vi "EN50160 Aggregation 10min.vi"(0 "voltage RMS values":dbl[](array[numeric]), 1 "fundamental voltage unbalance u2 [%]":dbl, 2 "voltage THD [%]":dbl[](array[numeric]), 3 "harmonic subgroups complex spectra":cluster{"f0":dbl, "df":dbl, "vectors":cdb[]}[](array[cluster]), 4 "system info in":refnum<class "EP System Info.lvclass">, 5 "error in (no error)":errorcluster, 6 "reset? (F)":bool, 7 "voltage flags? (F)":bool[](array[boolean]), 8 "data timestamp":timestamp) -> (14 "10min values":T1, 18 "system info out":refnum<class "EP System Info.lvclass">, 19 "error out":errorcluster)   [LabVIEW 2014, in "NI_EP_Power Quality.lvlib"]
doc: "Calculates aggregated values of power quality parameters for specific intervals. You use the aggregated values for further evaluations according to EN 50160:2007. The aggregation methods are compliant with Class S in IEC 61000-4-30:2008. The aggregation is based on a 10-cycle time interval for a 50 Hz power system or 12-cycle time interval for a 60 Hz power system. There is no overlap between aggregation intervals. This VI automatically restarts accumulation at the beginning of the next 10/12-cycle time interval after the previous interval expires. You must manually select the polymorphic instance you want to use.\n\nThis VI supports measuring single-bus single-line or multiple-bus single-line systems."
uses:
  <vilib>/addons/Electrical Power/PQ/NI_EP_Power Quality.lvlib
  <vilib>/addons/Electrical Power/PQ/Common/Classes/System Info/EP System Info.lvclass
  <vilib>/addons/Electrical Power/PQ/Common/Controls/ep_Aggregation Settings.ctl
  <vilib>/addons/Electrical Power/PQ/Aggregation/Custom Aggregation (1D DBL Array).vi
  <vilib>/addons/Electrical Power/PQ/Aggregation/Custom Aggregation (Deviation).vi
  <vilib>/addons/Electrical Power/PQ/Aggregation/Custom Aggregation (DBL).vi
  <vilib>/addons/Electrical Power/PQ/Aggregation/Custom Aggregation (Complex Spectra).vi
  <vilib>/addons/Electrical Power/PQ/Aggregation/Custom Aggregation (Flags).vi
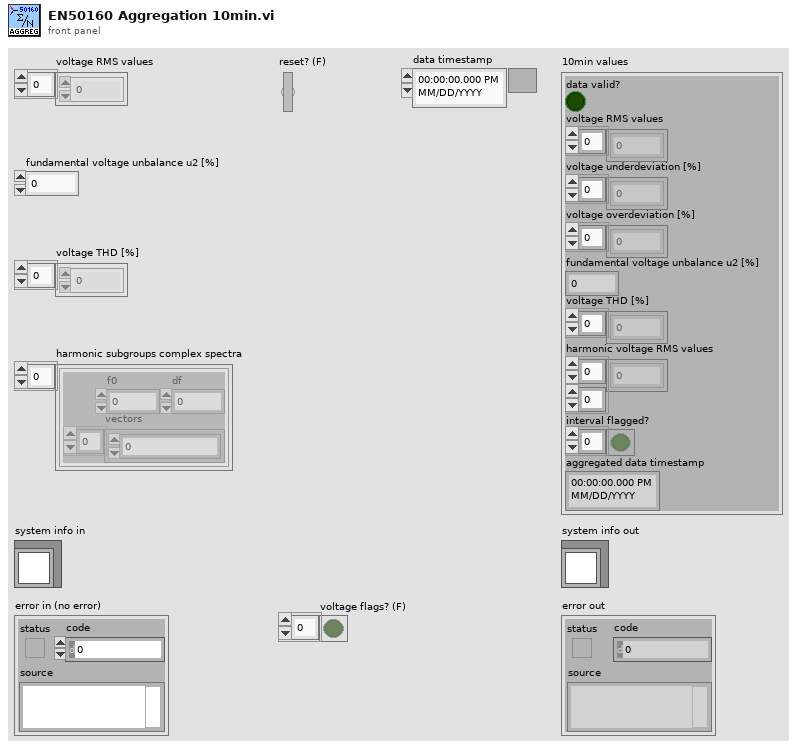
[diagram p1: front panel]
types:
  T1 = cluster{"data valid?":bool, "voltage RMS values":dbl[], "voltage underdeviation [%]":dbl[], "voltage overdeviation [%]":dbl[], "fundamental voltage unbalance u2 [%]  ":dbl, "voltage THD [%]":dbl[], "harmonic voltage RMS values":dbl[][], "interval flagged?":bool[], "aggregated data timestamp":timestamp}
  T2 = typedef "NI_EP_Power Quality.lvlib/ep_Aggregation Settings.ctl" = cluster{"interval":u32, "interval unit":enum16{"Runs", "Seconds", "Minutes", "Hours", "Days", "Weeks"}, "synchronization of intervals":enum16{"Not synchronized", "Interval rounded"}, "algorithm":enum16{"Average", "RMS"}}
  T3 = cluster{"f0":dbl, "df":dbl, "magnitudes":dbl[]}[]
  T4 = cluster{"aggregated data valid?":bool, "aggregated averaged/RMS values":dbl[], "Uunder [%]":dbl[], "Uover [%]":dbl[], "aggregated averaged/RMS value":dbl, "aggregated averaged/RMS values":dbl[], "magnitudes":dbl[][], "aggregated voltage flags":bool[], "aggregated data timestamp":timestamp}
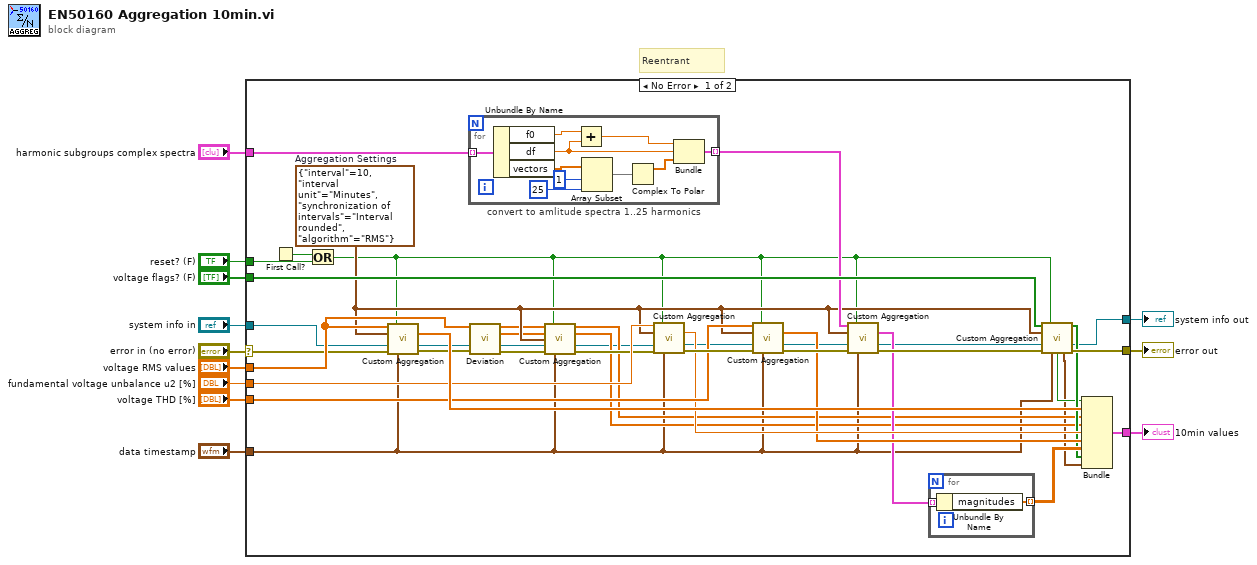
[diagram p0: block diagram]
diagram:
  # "Reentrant"
  n1 = case shown="No Error" "error in (no error)" {
    selector: "error in (no error)" -> [w24 w66]
    tunnel: "reset? (F)" -> [w35 _]
    tunnel: [w49 w66] -> w11
    tunnel: [w48 _] -> w10
    tunnel: "system info in" -> [w22 w65]
    tunnel: "voltage RMS values" -> [w34 _]
    tunnel: "fundamental voltage unbalance u2 [%]" -> [w45 _]
    tunnel: "voltage THD [%]" -> [w44 _]
    tunnel: "harmonic subgroups complex spectra" -> [w39 _]
    tunnel: "voltage flags? (F)" -> [w40 _]
    tunnel: "data timestamp" -> [w23 _]
    tunnel: [w15 w65] -> w2
    frame No Error {
      w30 = T2 {"interval"=10, "interval unit"=enum."Minutes", "synchronization of intervals"=enum."Interval rounded", "algorithm"=enum."RMS"}  # Aggregation Settings
      n2 = First Call?() -> (First Call?: T/F=w36:bool)
      n3 = Or(x=w36, y=w35) -> (x .or. y?=w27:bool)
      n4 = call-poly <vilib>:"Custom Aggregation.vi"("data in"=w34, "reset? (F)"=w27, "aggregation settings"=w30, "system info in"=w22, "error in (no error)"=w24, "data timestamp"=w23) -> ("aggregated averaged/RMS values"=w46:dbl[], "system info out"=w21:refnum<class "EP System Info.lvclass">, "error out"=w33:errorcluster)  [unwired: 3 in, 4 out]
      n5 = for "convert to amlitude spectra 1..25 harmonics" {
        tunnel: w39 -> [w62] mode=indexing
        tunnel: [w53] -> w38 mode=indexing
        n6 = Unbundle By Name(w62) -> ("f0"=w57:dbl, "df"=w55:dbl, "vectors"=w61:cdb[])
        n7 = Add(x=w57, y=w55) -> (x+y=w56:dbl)
        n8 = Array Subset(array=w61, index=1, length=25) -> (w60:cdb[])
        n9 = Complex To Polar(r * e^(i*theta)=w60) -> (r=w54:dbl[])  [unwired: 1 out]
        n10 = Bundle(w56, "df"=w55, w54) -> (w53:cluster{dbl, "df":dbl, dbl[]})  [unwired: 1 in]
      }
      n11 = call <vilib>:"Deviation.vi"("voltage RMS values"=w34, "system info in"=w21, "error in (no error)"=w33) -> ("Urms-under [V]"=w29:dbl[], "Urms-over [V]"=w28:dbl[], "system info out"=w20:refnum<class "EP System Info.lvclass">, "error out"=w32:errorcluster)  [unwired: 9 in]
      n12 = call-poly <vilib>:"Custom Aggregation.vi"("Urms-under [V]"=w29, "reset? (F)"=w27, "Urms-over [V]"=w28, "aggregation settings"=w30, "system info in"=w20, "error in (no error)"=w32, "data timestamp"=w23) -> ("Uunder [%]"=w26:dbl[], "Uover [%]"=w25:dbl[], "system info out"=w19:refnum<class "EP System Info.lvclass">, "error out"=w31:errorcluster)  [unwired: 3 in, 2 out]
      n13 = call-poly <vilib>:"Custom Aggregation.vi"("data in"=w45, "reset? (F)"=w27, "aggregation settings"=w30, "system info in"=w19, "error in (no error)"=w31, "data timestamp"=w23) -> ("aggregated averaged/RMS value"=w43:dbl, "system info out"=w18:refnum<class "EP System Info.lvclass">, "error out"=w52:errorcluster)  [unwired: 3 in, 4 out]
      n14 = call-poly <vilib>:"Custom Aggregation.vi"("data in"=w44, "reset? (F)"=w27, "aggregation settings"=w30, "system info in"=w18, "error in (no error)"=w52, "data timestamp"=w23) -> ("aggregated averaged/RMS values"=w42:dbl[], "system info out"=w17:refnum<class "EP System Info.lvclass">, "error out"=w51:errorcluster)  [unwired: 3 in, 4 out]
      n15 = call-poly <vilib>:"Custom Aggregation.vi"("complex spectra"=w38, "reset? (F)"=w27, "aggregation settings"=w30, "system info in"=w17, "error in (no error)"=w51, "data timestamp"=w23) -> ("aggregated averaged/RMS values"=w37:T3, "system info out"=w16:refnum<class "EP System Info.lvclass">, "error out"=w50:errorcluster)  [unwired: 3 in, 4 out]
      n16 = for {
        tunnel: w37 -> [w64] mode=indexing
        tunnel: [w63] -> w47 mode=indexing
        n17 = Unbundle By Name(w64) -> ("magnitudes"=w63:dbl[])
      }
      n18 = call-poly <vilib>:"Custom Aggregation.vi"("voltage flags? (F)"=w40, "reset? (F)"=w27, "aggregation settings"=w30, "system info in"=w16, "error in (no error)"=w50, "data timestamp"=w23) -> ("aggregated voltage flags"=w41:bool[], "system info out"=w15:refnum<class "EP System Info.lvclass">, "aggregated data valid?"=w14:bool, "aggregated data timestamp"=w13:timestamp, "error out"=w49:errorcluster)  [unwired: 5 in]
      n19 = Bundle("aggregated data valid?"=w14, "aggregated averaged/RMS values"=w46, "Uunder [%]"=w26, "Uover [%]"=w25, "aggregated averaged/RMS value"=w43, "aggregated averaged/RMS values"=w42, "magnitudes"=w47, "aggregated voltage flags"=w41, "aggregated data timestamp"=w13) -> (w48:T4)  [unwired: 1 in]
    }
    frame Error {
    }
  }
  "error out" <- w11
  "10min values" <- w10
  "system info out" <- w2
